vi "Name.vi"(11 "Numeric Data Type in":refnum<class "Numeric Data Type.lvclass">) -> (2 "String":string="Generic", 3 "Numeric Data Type (dup)":refnum<class "Numeric Data Type.lvclass">)   [LabVIEW 2018, in "Numeric Data Type.lvclass"]
uses:
  Numeric Data Type.lvclass
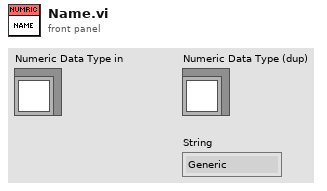
[diagram p1: front panel]
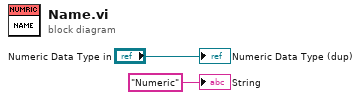
[diagram p0: block diagram]
diagram:
  "Numeric Data Type (dup)" <- "Numeric Data Type in"
  "String" <- "Numeric" ("String")
